vi "批量操作.vi"(8 "基路径":path=path "C:/Users/Administrator/Desktop/三菱MX模块测试/参数文档", 10 "Component Assemble Input":T1, 11 "input/output":bool) -> ()   [LabVIEW 2012]
uses:
  Component Assemble Input.ctl
  MX Operation Options.ctl
  <vilib>/Utility/file.llb/Read From Spreadsheet File (string).vi
panel:
  out "all rows":string[][](array[string]) caption="所有行"
  out "x-y":u32
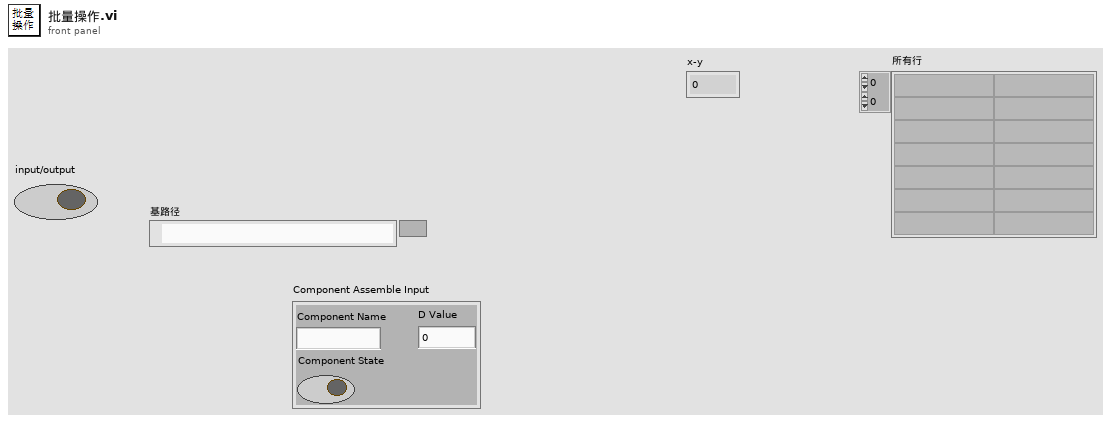
[diagram p1: front panel]
types:
  T1 = typedef "Component Assemble Input.ctl" = cluster{"Component Name":string, "Component State":bool, "D Value":dbl}
  T2 = typedef "MX Operation Options.ctl" = enum16{"MX Initial ", "MX Close", "Single component Read", "Single component Write", "Many component Read", "Many component Write", "Load Function Global"}
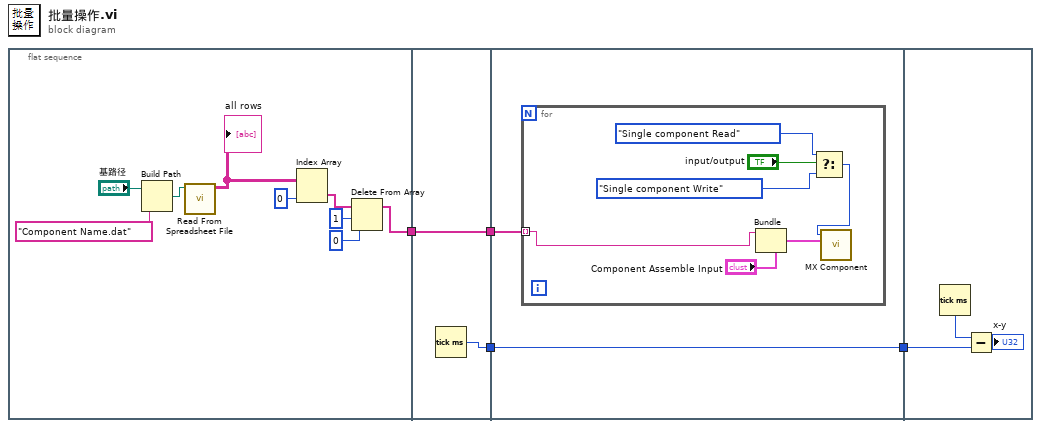
[diagram p0: block diagram]
diagram:
  n1 = flat-sequence {
    tunnel: [w5] -> w1
    tunnel: [w15] -> w4
    tunnel: [w14] -> w2
    tunnel: w1 -> [w14]
    tunnel: w4 -> [w17]
    tunnel: [w17] -> w3
    tunnel: w2 -> [w16]
    tunnel: w3 -> [w26]
    frame #0 {
      n2 = Build Path(base path="基路径", name or relative path="Component Name.dat" ("名称或相对路径")) -> (appended path=w8:path)
      n3 = call-poly <vilib>:"Read From Spreadsheet File.vi"("file path (dialog if empty)"=w8) -> ("all rows"=w9:string[][])  [unwired: 6 in, 4 out]
      "all rows" <- w9
      n4 = Index Array(array=w9, index (col)=0 ("禁用的索引 (列)")) -> (element=w11:string[])  [unwired: 1 in]
      n5 = Delete From Array(array=w11, length=1 ("长度"), index=0 ("索引")) -> (array with subset deleted=w5:string[])  [unwired: 1 out]
    }
    frame #1 {
      n6 = Tick Count (ms)() -> (millisecond timer value=w15:u32)
    }
    frame #2 {
      n7 = for {
        tunnel: w16 -> [w18] mode=indexing
        n8 = Bundle(cluster="Component Assemble Input", "Component Name"=w18) -> (w19:T1)  [unwired: 2 in]
        n9 = Select(t=MX_Operation_Options."Single component Read" ("MX Operation Options"), s="input/output", f=MX_Operation_Options."Single component Write" ("MX Operation Options")) -> (s? t:f=w24:T2)
        n10 = call "MX Component.vi"("Component Assemble Input"=w19, "MX Operation Options"=w24) -> ()  [unwired: 8 in, 2 out]
      }
    }
    frame #3 {
      n11 = Tick Count (ms)() -> (millisecond timer value=w27:u32)
      n12 = Subtract(x=w27, y=w26) -> (x-y=→"x-y":u32)
    }
  }
